vi "Build UI New Control.vi"(8 "error in (no error)":errorcluster, 11 "Panel Manager Controller.lvclass":refnum<class "Panel Manager Controller.lvclass">) -> (0 "error out":errorcluster, 3 "Panel Manager Controller.lvclass out":refnum<class "Panel Manager Controller.lvclass">)   [LabVIEW 2015, in "Panel Manager Controller.lvclass"]
uses:
  Panel Manager Controller.lvclass
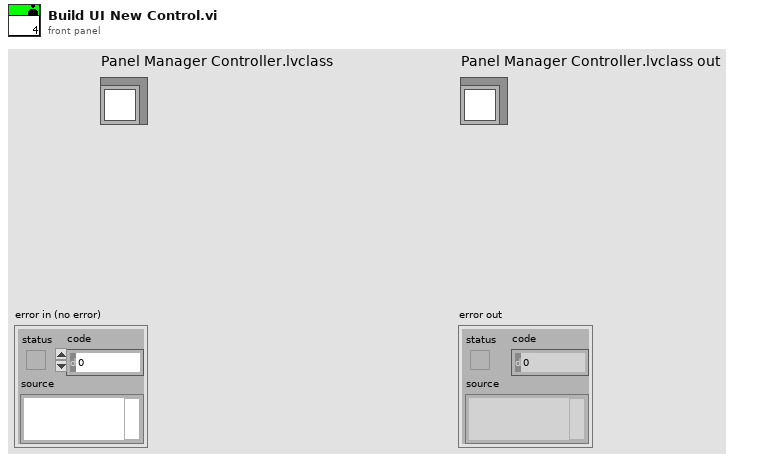
[diagram p1: front panel]
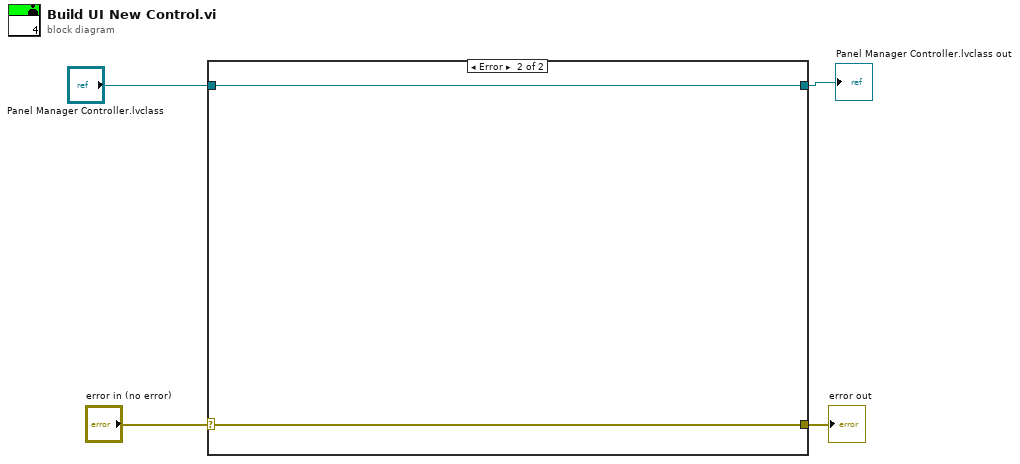
[diagram p0: block diagram]
diagram:
  n1 = case shown="Error" "error in (no error)" {
    selector: "error in (no error)" -> [w6 w8]
    tunnel: [w6 w8] -> w3
    tunnel: "Panel Manager Controller.lvclass" -> [w5 w7]
    tunnel: [w5 w7] -> w1
    frame No Error {
    }
    frame Error {
    }
  }
  "error out" <- w3
  "Panel Manager Controller.lvclass out" <- w1
